vi "DeSerializeInputs.vi"(0 "object in":refnum<class "Serializer.lvclass">, 2 "Inputtypes":variant[](array[variant]), 3 "InputString":string, 5 "error in (no error)":errorcluster) -> (14 "object out":refnum<class "Serializer.lvclass">, 16 "Inputs":variant[](array[variant]), 19 "error out":errorcluster)   [LabVIEW 2018, in "Serializer.lvclass"]
doc: "Deserialize the inputs string to an array of variants the set control value by index can handle.\nUse the input types as an layout for parsing the data if needed."
uses:
  Serializer.lvclass
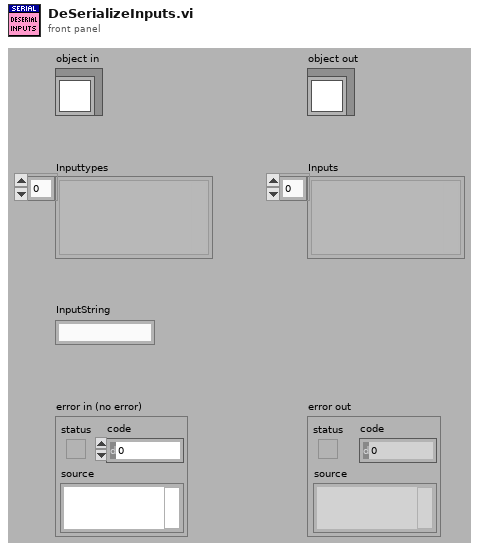
[diagram p1: front panel]
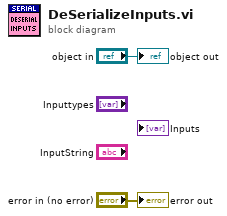
[diagram p0: block diagram]
diagram:
  "error out" <- "error in (no error)"
  "object out" <- "object in"
